vi "U Boat parse return string.vi"(0 "Return String":string) -> (1 "Tilt":dbl, 2 "Wind Speed":dbl, 3 "Wind Direction":dbl, 4 "Battery Volts":dbl)   [LabVIEW 2013]
doc: "This VI parses the return string from the U Boat Arbotix-M and presents sent values."
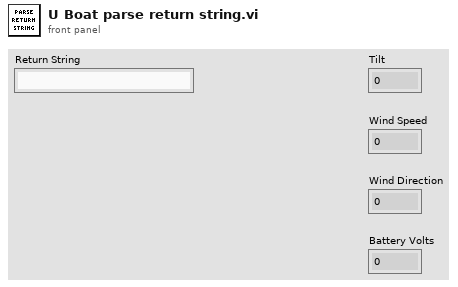
[diagram p1: front panel]
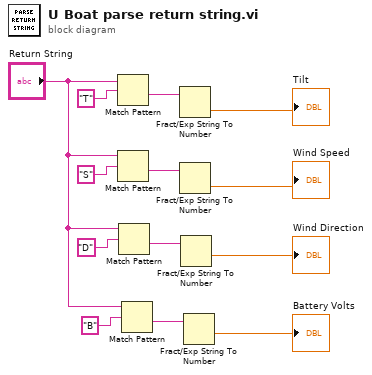
[diagram p0: block diagram]
diagram:
  n1 = Match Pattern(string="Return String", regular expression="T") -> (after substring=w12:string)  [unwired: 1 in, 3 out]
  n2 = Match Pattern(string="Return String", regular expression="S") -> (after substring=w9:string)  [unwired: 1 in, 3 out]
  n3 = Match Pattern(string="Return String", regular expression="D") -> (after substring=w6:string)  [unwired: 1 in, 3 out]
  n4 = Match Pattern(string="Return String", regular expression="B") -> (after substring=w3:string)  [unwired: 1 in, 3 out]
  n5 = Fract/Exp String To Number(string=w12) -> (number=→"Tilt":dbl)  [unwired: 3 in, 1 out]
  n6 = Fract/Exp String To Number(string=w9) -> (number=→"Wind Speed":dbl)  [unwired: 3 in, 1 out]
  n7 = Fract/Exp String To Number(string=w6) -> (number=→"Wind Direction":dbl)  [unwired: 3 in, 1 out]
  n8 = Fract/Exp String To Number(string=w3) -> (number=→"Battery Volts":dbl)  [unwired: 3 in, 1 out]
